vi "TPNT_TP2Str.vi"(6 "device":string, 9 "index in":i32, 10 "TestPoint In":T1={"name"="", "type"="", "algor"=[], "update_rate"=0.0, "Limits"={"Alarm Type"="", "Lower "=0.0, "Upper"=0.0, "Nominal"=0.0, "outrange"=FALSE, "Check"=TRUE, "latch"=FALSE, "level"=""}, "Samples"={"samples"=0, "counter"=0, "Values"=[], "Current Value"="", "filter"="", "precision"=2}, "next_update"=0, "Status"="", "monitor"=TRUE, "error"=FALSE, "Log"={"log"=FALSE, "file"=path "", "type"="", "format"="", "updaterate"=0.0, "nex_update"=0, "mode"=""}, "permissions"="", "ID"=""} {"Log"."updaterate" format="%.2f"; "Samples"."Values" format="%.2f"; "Samples"."samples" min=1 step=1; "Limits"."Nominal" format="%.2f"; "Limits"."Upper" format="%.2f"; "Limits"."Lower" format="%.2f"; "update_rate" format="%.2f"}) -> (2 "TP out":string)   [LabVIEW 2016]
uses:
  TPNT_TP.ctl
  TPNT_Limits.ctl
  TPNT_Samples.ctl
  TPNT_Log.ctl
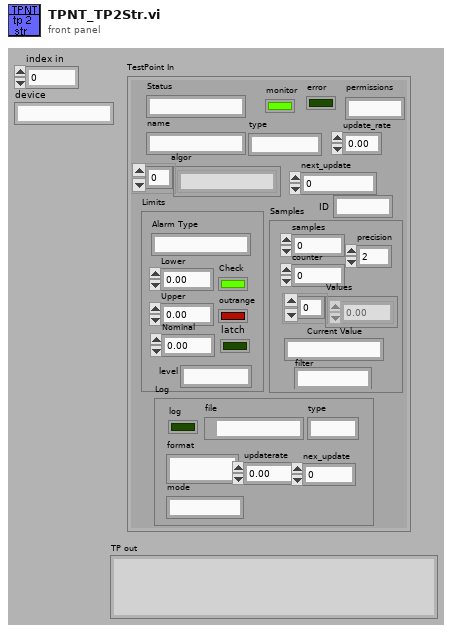
[diagram p1: front panel]
types:
  T1 = typedef "TPNT_TP.ctl" = cluster{"name":string, "type":string, "algor":string[], "update_rate":sgl, "Limits":T2, "Samples":T3, "next_update":u32, "Status":string, "monitor":bool, "error":bool, "Log":T4, "permissions":string, "ID":string}
  T2 = typedef "TPNT_Limits.ctl" = cluster{"Alarm Type":string, "Lower ":dbl, "Upper":dbl, "Nominal":dbl, "outrange":bool, "Check":bool, "latch":bool, "level":string}
  T3 = typedef "TPNT_Samples.ctl" = cluster{"samples":i32, "counter":i32, "Values":dbl[], "Current Value":string, "filter":string, "precision":u8}
  T4 = typedef "TPNT_Log.ctl" = cluster{"log":bool, "file":path, "type":string, "format":string, "updaterate":dbl, "nex_update":u32, "mode":string}
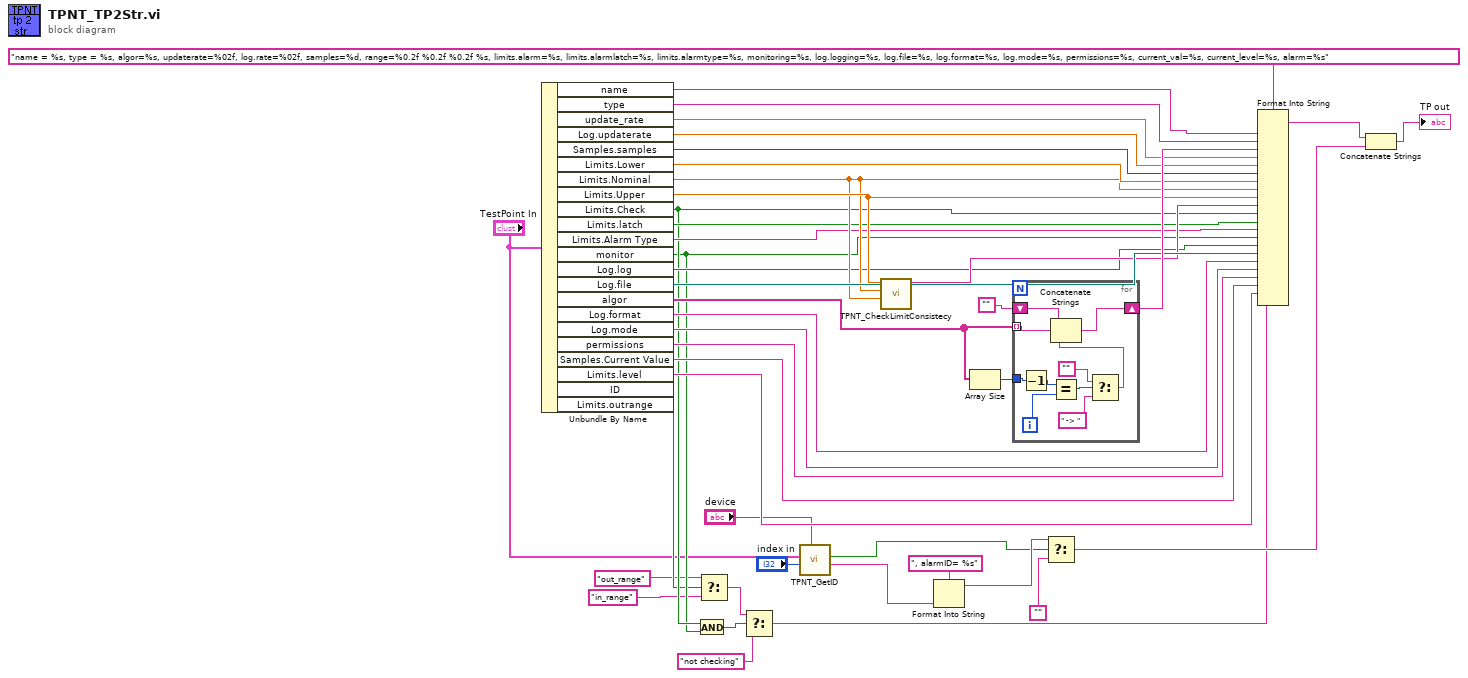
[diagram p0: block diagram]
diagram:
  n1 = Unbundle By Name("TestPoint In") -> ("name"=w42:string, "type"=w41:string, "update_rate"=w36:sgl, "Log.updaterate"=w35:dbl, "Samples.samples"=w34:i32, "Limits.Lower"=w33:dbl, "Limits.Nominal"=w30:dbl, "Limits.Upper"=w31:dbl, "Limits.Check"=w16:bool, "Limits.latch"=w27:bool, "Limits.Alarm Type"=w24:string, "monitor"=w13:bool, "Log.log"=w28:bool, "Log.file"=w32:path, "algor"=w39:string[], "Log.format"=w26:string, "Log.mode"=w25:string, "permissions"=w23:string, "Samples.Current Value"=w22:string, "Limits.level"=w21:string, "Limits.outrange"=w12:bool)  [unwired: 1 out]
  n2 = And(x=w16, y=w13) -> (x .and. y?=w14:bool)
  n3 = Select(t="out_range", s=w12, f="in_range") -> (s? t:f=w9:string)
  n4 = Select(t=w9, s=w14, f="not checking") -> (s? t:f=w8:string)
  n5 = call "TPNT_GetID.vi"("device"="device", "index in"="index in", "testpoint In"="TestPoint In") -> ("id out"=w5:string, "id?"=w2:bool)  [unwired: 7 out]
  n6 = call "TPNT_CheckLimitConsistecy.vi"("lower"=w30, "nominal"=w30, "upper"=w31) -> ("message"=w29:string)  [unwired: 1 in, 7 out]
  n7 = Format Into String(format string=", alarmID= %s", w5) -> (resulting string=w3:string)  [unwired: 2 in, 1 out]
  n8 = Array Size(array=w39) -> (size(s)=w38:i32)
  n9 = for {
    tunnel: w39 -> [w53] mode=indexing
    shift-right: [w52] -> w37
    shift-left: "" -> [w51]
    tunnel: w38 -> [w50]
    i -> [w48]
    n10 = Decrement(x=w50) -> (x-1=w49:i32)
    n11 = Equal?(x=w49, y=w48) -> (x = y?=w47:bool)
    n12 = Select(t="", s=w47, f=" -> ") -> (s? t:f=w44:string)
    n13 = Concatenate Strings(w51, w53, w44) -> (w52:string)
  }
  n14 = Select(t=w3, s=w2, f="") -> (s? t:f=w18:string)
  n15 = Format Into String(format string="name = %s, type = %s, algor=%s, updaterate=%02f, log.rate=%02f, samples=%d, range=%0.2f %0.2f %0.2f %s, limits.alarm=%s, limits.alarmlatch=%s, limits.alarmtype=%s, monitoring=%s, log.logging=%s, log.file=%s, log.format=%s, log.mode=%s, permissions=%s, current_val=%s, current_level=%s, alarm=%s", w42, w41, w37, w36, w35, w34, w33, w30, w31, w29, w16, w27, w24, w13, w28, w32, w26, w25, w23, w22, w21, w8) -> (resulting string=w19:string)  [unwired: 2 in, 1 out]
  n16 = Concatenate Strings(w19, w18) -> (→"TP out":string)
